vi "Get Feature Representation.vi"(8 "error in (no error)":errorcluster, 10 "Feature":string, 11 "Camera in":refnum<class "Camera.lvclass">) -> (0 "error out":errorcluster, 2 "Representation":T1, 3 "Camera":refnum<class "Camera.lvclass">)   [LabVIEW 2020, in "Camera.lvclass"]
uses:
  Camera.lvclass
  Camera.lvclass/Camera.ctl
  bin/gindustrialcam_32-1.dll
  Representation.ctl
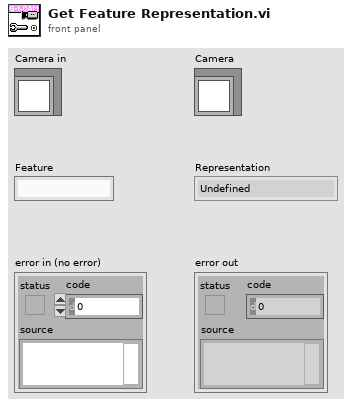
[diagram p1: front panel]
types:
  T1 = typedef "Camera.lvclass/Representation.ctl" = enum8{"Undefined", "Linear", "Logarithmic", "Boolean", "Pure Number", "Hex Number", "IP Address", "MAC Address"}
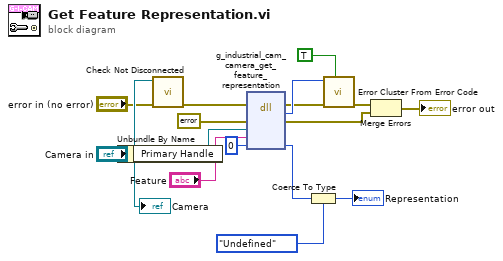
[diagram p0: block diagram]
diagram:
  n1 = Unbundle By Name("Camera in") -> ("Primary Handle"=w12:refnum<data-value>)
  n2 = call "Check Not Disconnected.vi"("error in (no error)"="error in (no error)", "Camera in"="Camera in") -> ("error out"=w13:errorcluster)  [unwired: 9 in]
  n3 = dll-call lib="C:/serenial/lib/g-industrial-camera/LabVIEW/g_industrial_cam/bin/gindustrialcam_*-1.*" fn="g_industrial_cam_camera_get_feature_representation"(error in=w13, "err"=errorcluster {"status"=FALSE, "code"=0, "source"=""} ("error constant"), "edvr"=w12, "feature"="Feature", "representation"=u8 0) -> (error out=w6:errorcluster, "Mg_Error"=w7:i32, "err"=w9:errorcluster, "representation"=w3:u8)  [unwired: 4 in, 1 out]
  n4 = Coerce To Type(0:w3, 1:Representation."Undefined" ("Representation")) -> (2:→"Representation":T1)
  n5 = call <vilib>:"Error Cluster From Error Code.vi"("show call chain? (False)"=TRUE, "error in (no error)"=w6, "error code (0)"=w7) -> ("error out"=w8:errorcluster)  [unwired: 6 in]
  n6 = Merge Errors(w8, w9) -> (→"error out":errorcluster)
  "Camera" <- "Camera in"
